vi "Control_from_Kiearn.vi"() -> ()   [LabVIEW 2015]
panel:
  in  "Set bias":string
  in  "Set frequency":string
  out "Average time":string
  in  "Set average time":string
  in  "Set voltage":string
  out "Bias":string
  out "Frequency":string
  out "Voltage":string
  in  "Measurement ON/OFF":bool
  out "Meaurement results":string
  in  "Record new values":bool
  in  "error in (no error)":errorcluster
  out "error out":errorcluster
  # "NOTE: Bias has only three options ILOW, IHIGH and OFF"
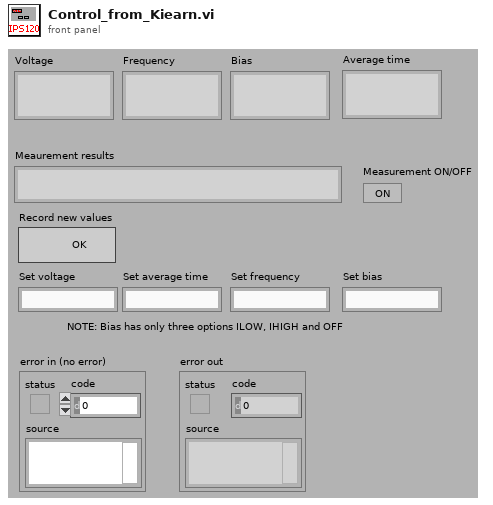
[diagram p1: front panel]
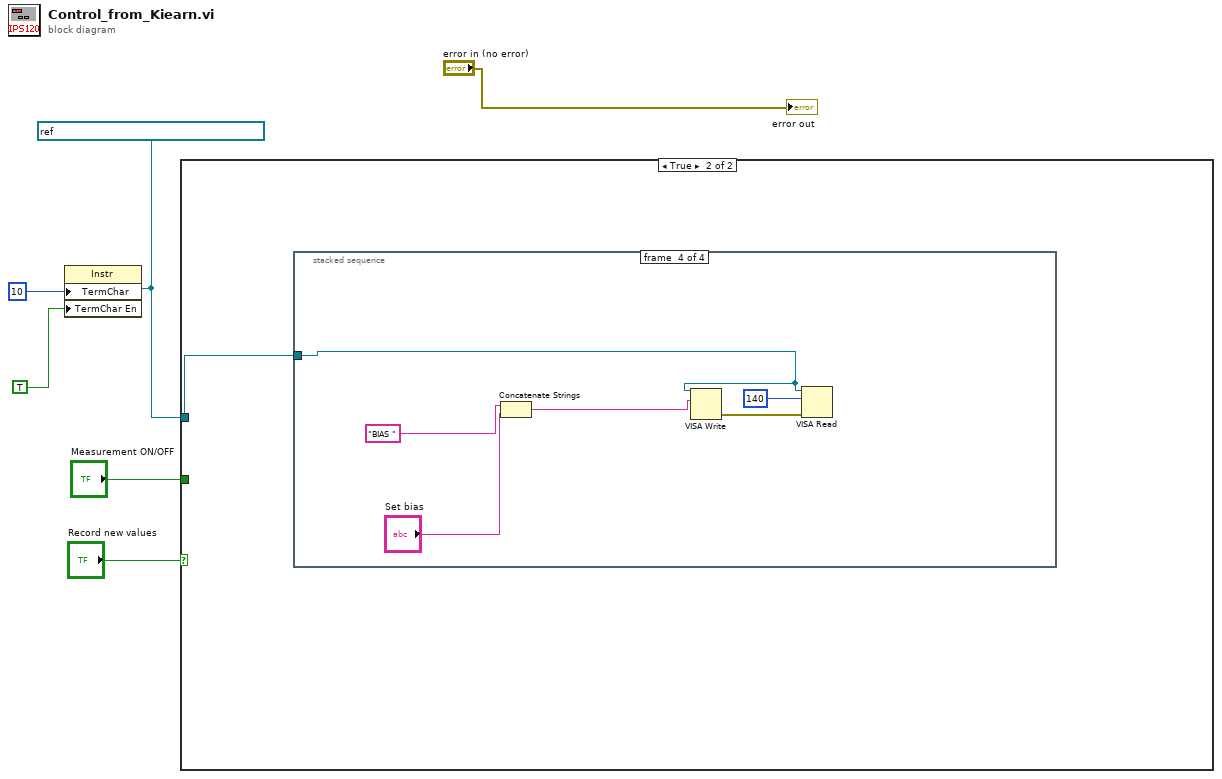
[diagram p0: block diagram]
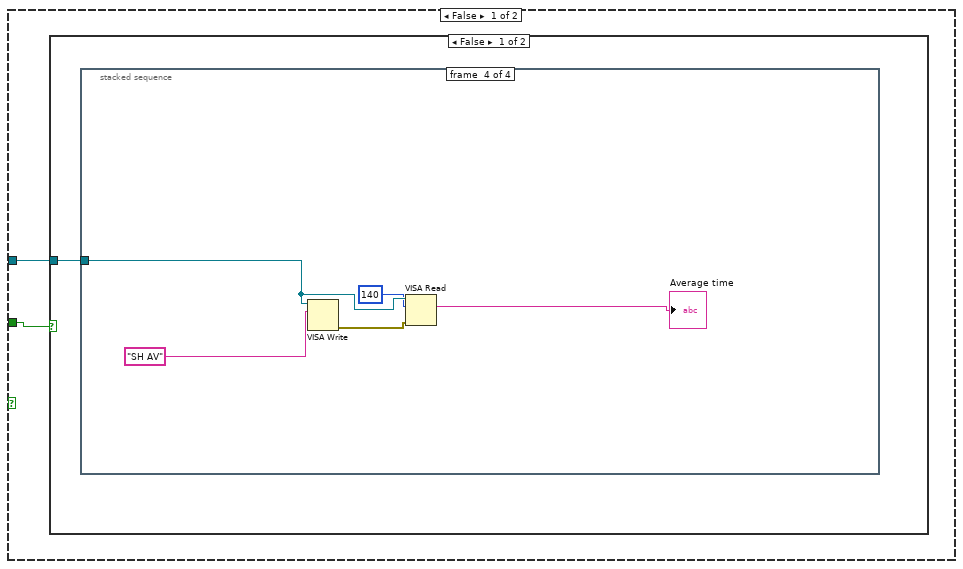
[diagram p2: hidden frame]
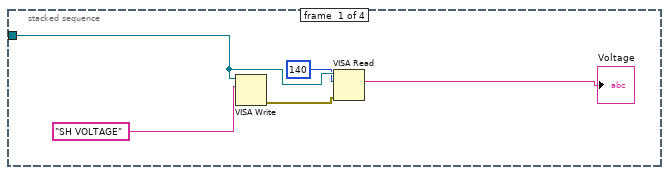
[diagram p3: hidden frame]
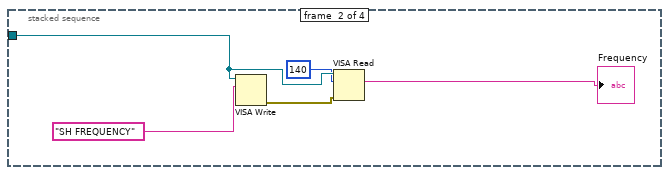
[diagram p4: hidden frame]
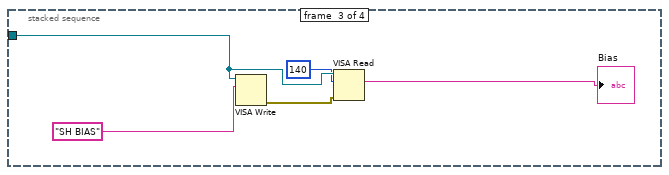
[diagram p5: hidden frame]
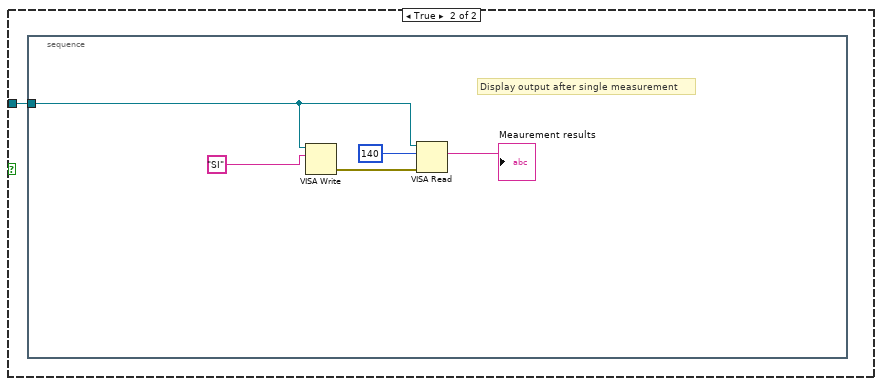
[diagram p6: hidden frame]
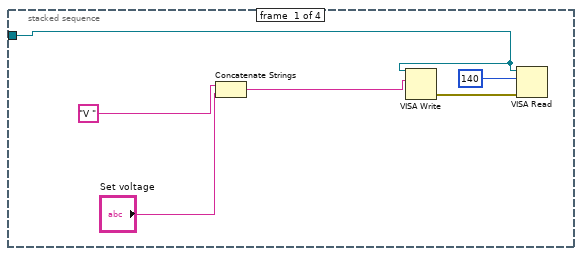
[diagram p7: hidden frame]
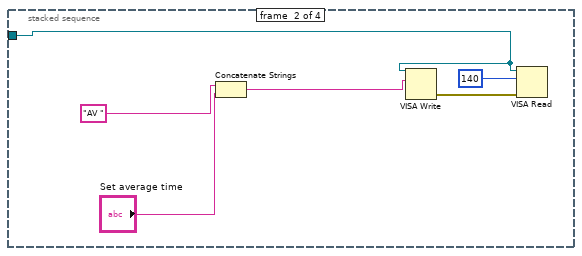
[diagram p8: hidden frame]
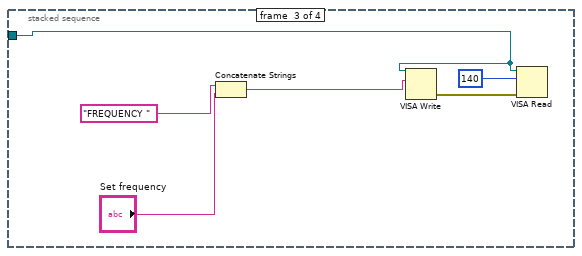
[diagram p9: hidden frame]
diagram:
  w3 = refnum<visa-resource-name> "GPIB0::28::INSTR" ("VISA resource name")
  n1 = property class="Instr"(reference=w3, "TermChar"=10, "TermChar En"=TRUE) -> ()  [unwired: 1 in, 2 out]
  n2 = case shown="True" "Record new values" {
    tunnel: w3 -> [w8 w36]
    tunnel: "Measurement ON/OFF" -> [w7 _]
    frame False {
      n3 = case shown="False" w7 {
        tunnel: w8 -> [w9 w30]
        frame False {
          n4 = stacked-sequence {
            tunnel: w9 -> [w14 w19 w24 w29]
            frame #0 {
              n5 = VISA Write(VISA resource name=w14, write buffer="SH VOLTAGE") -> (error out=w12:errorcluster)  [unwired: 1 in, 2 out]
              n6 = VISA Read(VISA resource name=w14, byte count=140, error in (no error)=w12) -> (read buffer=→"Voltage":string)  [unwired: 3 out]
            }
            frame #1 {
              n7 = VISA Write(VISA resource name=w19, write buffer="SH FREQUENCY") -> (error out=w17:errorcluster)  [unwired: 1 in, 2 out]
              n8 = VISA Read(VISA resource name=w19, byte count=140, error in (no error)=w17) -> (read buffer=→"Frequency":string)  [unwired: 3 out]
            }
            frame #2 {
              n9 = VISA Write(VISA resource name=w24, write buffer="SH BIAS") -> (error out=w22:errorcluster)  [unwired: 1 in, 2 out]
              n10 = VISA Read(VISA resource name=w24, byte count=140, error in (no error)=w22) -> (read buffer=→"Bias":string)  [unwired: 3 out]
            }
            frame #3 {
              n11 = VISA Write(VISA resource name=w29, write buffer="SH AV") -> (error out=w27:errorcluster)  [unwired: 1 in, 2 out]
              n12 = VISA Read(VISA resource name=w29, byte count=140, error in (no error)=w27) -> (read buffer=→"Average time":string)  [unwired: 3 out]
            }
          }
        }
        frame True {
          n13 = stacked-sequence {
            tunnel: w30 -> [w33]
            frame #0 {
              # "Display output after single measurement"
              n14 = VISA Write(VISA resource name=w33, write buffer="SI" ("string")) -> (error out=w35:errorcluster)  [unwired: 1 in, 2 out]
              n15 = VISA Read(VISA resource name=w33, byte count=140, error in (no error)=w35) -> (read buffer=→"Meaurement results":string)  [unwired: 3 out]
            }
          }
        }
      }
    }
    frame True {
      n16 = stacked-sequence {
        tunnel: w36 -> [w40 w46 w52 w58]
        frame #0 {
          n17 = Concatenate Strings("V ", "Set voltage") -> (w39:string)
          n18 = VISA Write(VISA resource name=w40, write buffer=w39) -> (error out=w42:errorcluster)  [unwired: 1 in, 2 out]
          n19 = VISA Read(VISA resource name=w40, byte count=140, error in (no error)=w42) -> ()  [unwired: 4 out]
        }
        frame #1 {
          n20 = Concatenate Strings("AV ", "Set average time") -> (w45:string)
          n21 = VISA Write(VISA resource name=w46, write buffer=w45) -> (error out=w48:errorcluster)  [unwired: 1 in, 2 out]
          n22 = VISA Read(VISA resource name=w46, byte count=140, error in (no error)=w48) -> ()  [unwired: 4 out]
        }
        frame #2 {
          n23 = Concatenate Strings("FREQUENCY ", "Set frequency") -> (w51:string)
          n24 = VISA Write(VISA resource name=w52, write buffer=w51) -> (error out=w54:errorcluster)  [unwired: 1 in, 2 out]
          n25 = VISA Read(VISA resource name=w52, byte count=140, error in (no error)=w54) -> ()  [unwired: 4 out]
        }
        frame #3 {
          n26 = Concatenate Strings("BIAS ", "Set bias") -> (w57:string)
          n27 = VISA Write(VISA resource name=w58, write buffer=w57) -> (error out=w60:errorcluster)  [unwired: 1 in, 2 out]
          n28 = VISA Read(VISA resource name=w58, byte count=140, error in (no error)=w60) -> ()  [unwired: 4 out]
        }
      }
    }
  }
  "error out" <- "error in (no error)"
